vi "Query Keys Wrapper.vi"(8 "error in (no error)":errorcluster, 9 "timeout_ms":u64=2000, 10 "key_expr":string, 11 "Reader Handle":u64) -> (0 "error out":errorcluster, 3 "Query Key Return":T1 {"Data Bytes" format="%.0x"; "Key Bytes" format="%.0x"})   [LabVIEW 2021, in "Zenoh.lvclass"]
uses:
  Zenoh.lvclass
  typedef/Query Keys Return.ctl
  typedef/Zenoh Errors.ctl
  <vilib>/CIF Foundation/CIF Utilities/Errors/Append Error Location.vi
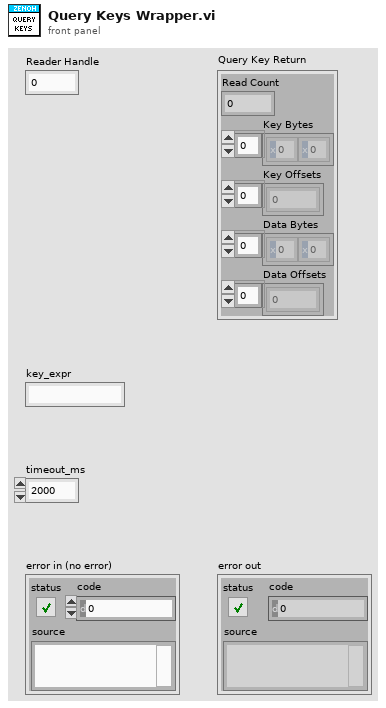
[diagram p1: front panel]
types:
  T1 = typedef "Zenoh.lvclass/Query Keys Return.ctl" = cluster{"Read Count":i32, "Key Bytes":u8[], "Key Offsets":u32[], "Data Bytes":u8[], "Data Offsets":u32[]}
  T2 = typedef "Zenoh.lvclass/Zenoh Errors.ctl" = enum16{"Open Session Error", "Open Subscription Error", "Declare Liveliness", "Query Keys"}
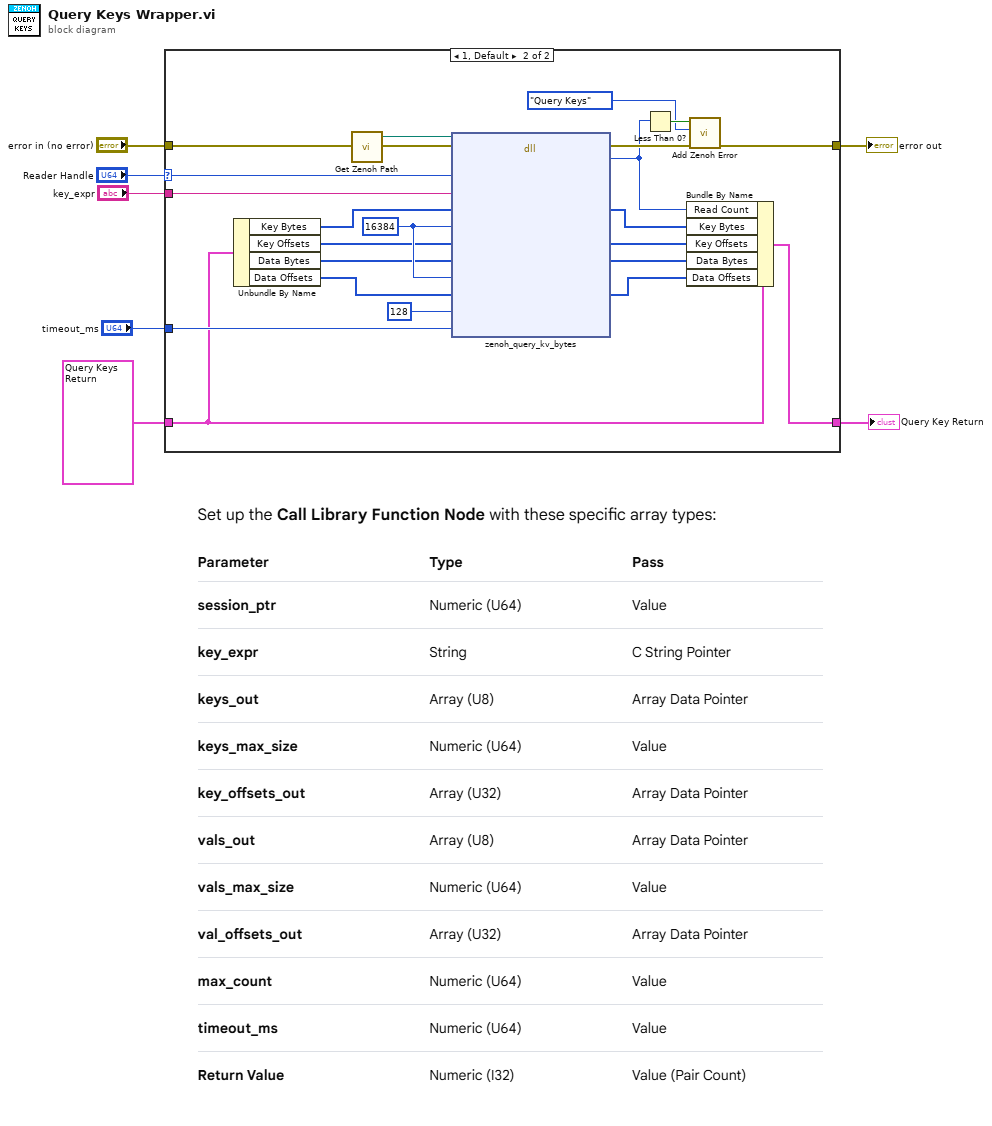
[diagram p0: block diagram]
diagram:
  n1 = case shown="1, Default" "Reader Handle" {
    selector: "Reader Handle" -> [_ w30]
    tunnel: [w9 w22] -> w7
    tunnel: "error in (no error)" -> [w9 w31]
    tunnel: "key_expr" -> [_ w28]
    tunnel: "timeout_ms" -> [_ w27]
    tunnel: T1 {"Read Count"=0, "Key Bytes"=array[16384 elements], "Key Offsets"=[0, 0, 0, 0, 0, 0, 0, 0, 0, 0, 0, 0, 0, 0, 0, 0, 0, 0, 0, 0, 0, 0, 0, 0, 0, 0, 0, 0, 0, 0, 0, 0, 0, 0, 0, 0, 0, 0, 0, 0, 0, 0, 0, 0, 0, 0, 0, 0, 0, 0, 0, 0, 0, 0, 0, 0, 0, 0, 0, 0, 0, 0, 0, 0, 0, 0, 0, 0, 0, 0, 0, 0, 0, 0, 0, 0, 0, 0, 0, 0, 0, 0, 0, 0, 0, 0, 0, 0, 0, 0, 0, 0, 0, 0, 0, 0, 0, 0, 0, 0, 0, 0, 0, 0, 0, 0, 0, 0, 0, 0, 0, 0, 0, 0, 0, 0, 0, 0, 0, 0, 0, 0, 0, 0, 0, 0, 0, 0], "Data Bytes"=array[16384 elements], "Data Offsets"=[0, 0, 0, 0, 0, 0, 0, 0, 0, 0, 0, 0, 0, 0, 0, 0, 0, 0, 0, 0, 0, 0, 0, 0, 0, 0, 0, 0, 0, 0, 0, 0, 0, 0, 0, 0, 0, 0, 0, 0, 0, 0, 0, 0, 0, 0, 0, 0, 0, 0, 0, 0, 0, 0, 0, 0, 0, 0, 0, 0, 0, 0, 0, 0, 0, 0, 0, 0, 0, 0, 0, 0, 0, 0, 0, 0, 0, 0, 0, 0, 0, 0, 0, 0, 0, 0, 0, 0, 0, 0, 0, 0, 0, 0, 0, 0, 0, 0, 0, 0, 0, 0, 0, 0, 0, 0, 0, 0, 0, 0, 0, 0, 0, 0, 0, 0, 0, 0, 0, 0, 0, 0, 0, 0, 0, 0, 0, 0]} ("Query Key Return 2") -> [w8 w16]
    tunnel: [w8 w10] -> w1
    frame 0 {
    }
    frame 1, Default {
      w26 = u64 16384 ("max_buffer_size")
      n2 = Unbundle By Name(w16) -> ("Key Bytes"=w20:u8[], "Key Offsets"=w18:u32[], "Data Bytes"=w19:u8[], "Data Offsets"=w17:u32[])
      n3 = call "Get Zenoh Path.vi"() -> ("Library Path"=w29:path)  [unwired: 4 in]
      n4 = dll-call lib="C:/Program Files/CIF_Foundation/Libraries/zenoh_lv_wrapper.dll" fn="zenoh_query_kv_bytes"(path in=w29, error in=w31, "session_ptr"=w30, "key_expr"=w28, "keys_out"=w20, "keys_max_size"=w26, "key_offsets_out"=w18, "vals_out"=w19, "vals_max__size"=w26, "val_offsets_out"=w17, "max_count"=u64 128, "timeout_ms"=w27) -> (error out=w21:errorcluster, "return type"=w15:i32, "keys_out"=w14:u8[], "key_offsets_out"=w13:u32[], "vals_out"=w12:u8[], "val_offsets_out"=w11:u32[])  [unwired: 7 in, 1 out]
      n5 = Less Than 0?(x=w15) -> (x < 0?=w24:bool)
      n6 = Bundle By Name(cluster=w16, "Read Count"=w15, "Key Bytes"=w14, "Key Offsets"=w13, "Data Bytes"=w12, "Data Offsets"=w11) -> (w10:T1)
      n7 = call "Add Zenoh Error.vi"("error in (no error)"=w21, "Error"=Zenoh_Errors."Query Keys", "Insert Error"=w24) -> ("error out"=w22:errorcluster)  [unwired: 8 in]
    }
  }
  "error out" <- w7
  "Query Key Return" <- w1
